vi "Signal Append.vi"() -> ()   [LabVIEW 2013]
panel:
  out "Flow":dynamicdata(graph)
  out "Audio":dynamicdata(graph)
  out "Pressure":dynamicdata(graph)
  out "Full Graph":dynamicdata(graph)
  out "SPL":dynamicdata(graph)
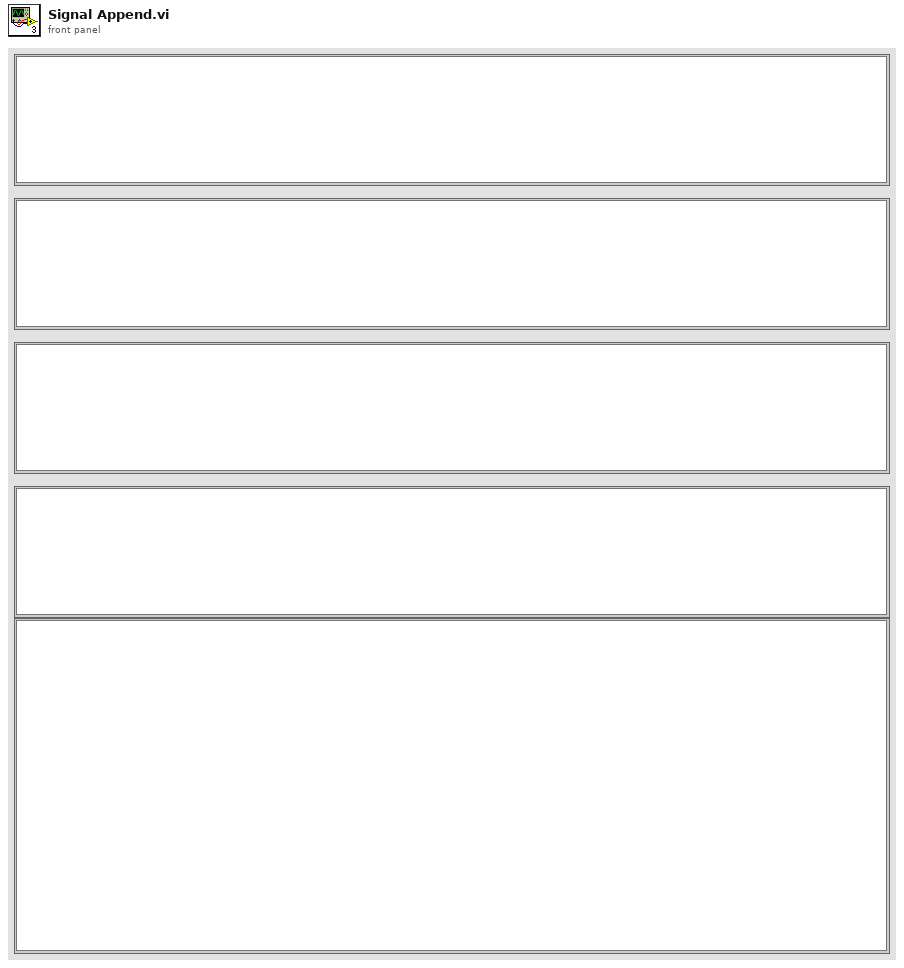
[diagram p1: front panel]
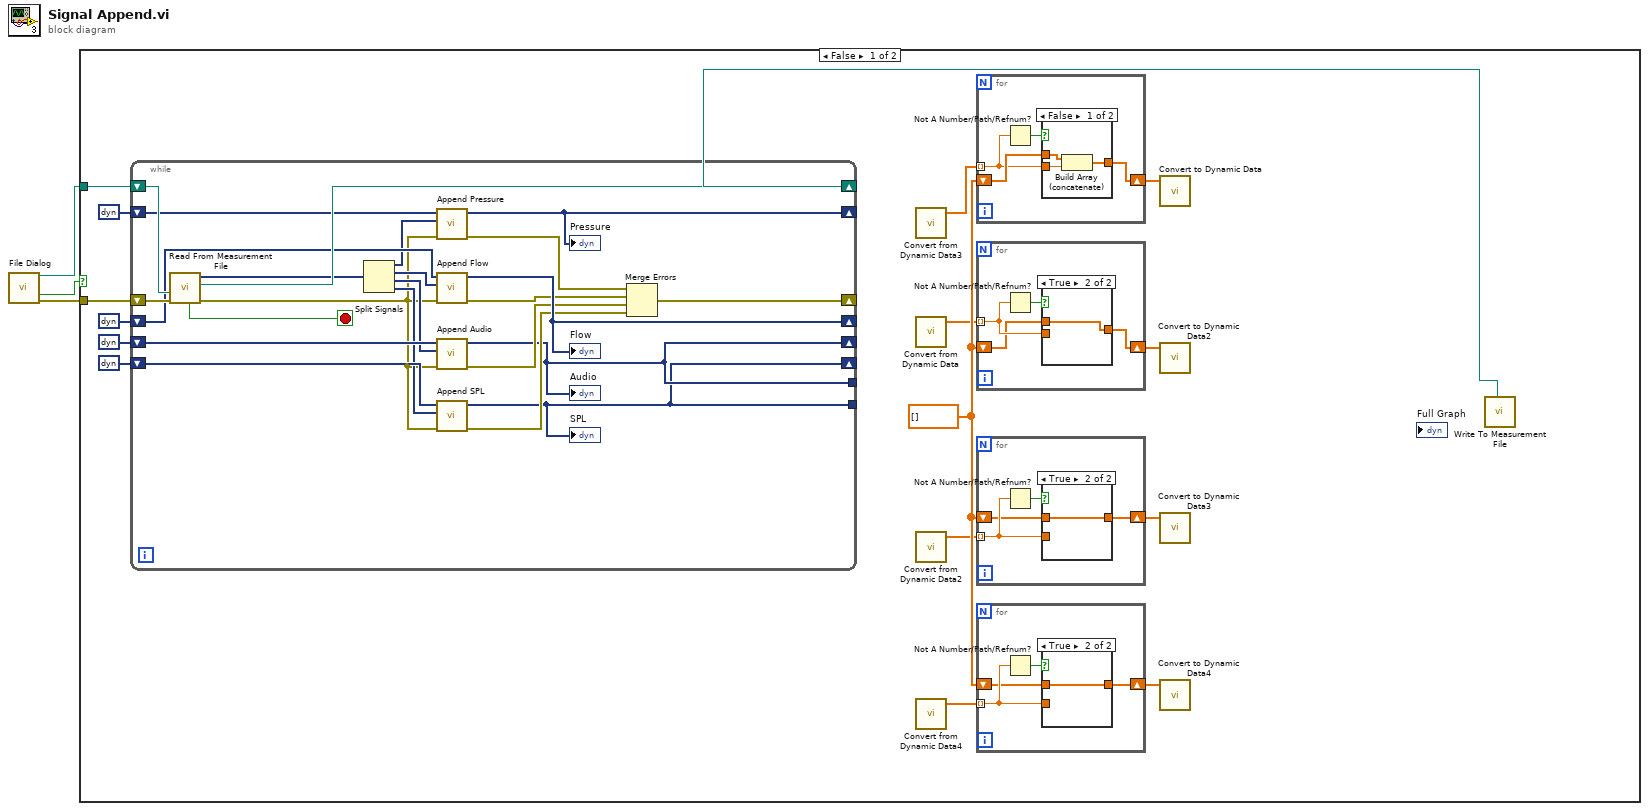
[diagram p0: block diagram]
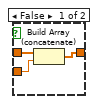
[diagram p2: hidden frame]
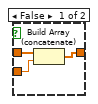
[diagram p3: hidden frame]
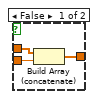
[diagram p4: hidden frame]
diagram:
  n1 = call "File Dialog"() -> ("selected path"=w3:path, "cancelled"=w1:bool, "error out"=w2:errorcluster)  [unwired: 12 in, 1 out]
  n2 = case shown="False" w1 {
    tunnel: w3 -> [w19 _]
    tunnel: w2 -> [w18 _]
    frame False {
      w7 = dbl[] [] ("Arrayin 2")
      n3 = while {
        shift-right: [w60] -> _
        shift-left: w18 -> [w73]
        shift-right: [w74] -> w13
        shift-left: w19 -> [w72]
        shift-right: [w63] -> _
        shift-left: dynamicdata [] ("Waveform Graph") -> [w70]
        shift-right: [w62] -> _
        shift-left: dynamicdata [] ("Waveform Graph") -> [w69]
        shift-right: [w53] -> _
        shift-left: dynamicdata [] ("Waveform Graph") -> [w68]
        shift-right: [w52] -> _
        shift-left: dynamicdata [] ("Waveform Graph") -> [w67]
        tunnel: [w53] -> _
        tunnel: [w52] -> _
        stop <- w71 stop-if-true
        n4 = call "Read From Measurement File"("error in (no error)"=w73, "Filename"=w72) -> ("error out"=w55:errorcluster, "Filename Out"=w74:path, "Signals"=w54:dynamicdata, "EOF?"=w71:bool)  [unwired: 4 in, 2 out]
        n5 = Split Signals(w54) -> (w66:dynamicdata, w65:dynamicdata, w64:dynamicdata, w61:dynamicdata)  [unwired: 4 in]
        n6 = call "Append Pressure"("error in (no error)"=w55, "Input Signal B"=w66, "Input Signal A"=w70) -> ("error out"=w59:errorcluster, "Appended Signals"=w63:dynamicdata)  [unwired: 7 in]
        "Pressure" <- w63
        n7 = call "Append Flow"("error in (no error)"=w55, "Input Signal B"=w65, "Input Signal A"=w69) -> ("error out"=w58:errorcluster, "Appended Signals"=w62:dynamicdata)  [unwired: 7 in]
        "Flow" <- w62
        n8 = call "Append Audio"("error in (no error)"=w55, "Input Signal B"=w64, "Input Signal A"=w68) -> ("error out"=w57:errorcluster, "Appended Signals"=w53:dynamicdata)  [unwired: 7 in]
        "Audio" <- w53
        n9 = call "Append SPL"("error in (no error)"=w55, "Input Signal B"=w61, "Input Signal A"=w67) -> ("error out"=w56:errorcluster, "Appended Signals"=w52:dynamicdata)  [unwired: 7 in]
        "SPL" <- w52
        n10 = Merge Errors(w59, w58, w57, w56) -> (w60:errorcluster)
      }
      n11 = call "Convert from Dynamic Data3"() -> ("Array"=w12:dbl[])  [unwired: 4 in]
      n12 = call "Convert from Dynamic Data"() -> ("Array"=w6:dbl[])  [unwired: 4 in]
      n13 = call "Convert from Dynamic Data2"() -> ("Array"=w5:dbl[])  [unwired: 4 in]
      n14 = call "Convert from Dynamic Data4"() -> ("Array"=w4:dbl[])  [unwired: 4 in]
      n15 = for {
        tunnel: w12 -> [w44] mode=indexing
        shift-right: [w45] -> w11
        shift-left: w7 -> [w46]
        n16 = Not A Number/Path/Refnum?(number/path/refnum=w44) -> (NaN/Path/Refnum?=w47:bool)
        n17 = case shown="False" w47 {
          tunnel: w46 -> [w50 w51]
          tunnel: [w49 w51] -> w45
          tunnel: w44 -> [w48 _]
          frame False {
            n18 = Build Array (concatenate)(w50, w48) -> (w49:dbl[])
          }
          frame True {
          }
        }
      }
      n19 = for {
        tunnel: w6 -> [w38] mode=indexing
        shift-right: [w36] -> w10
        shift-left: w7 -> [w37]
        n20 = Not A Number/Path/Refnum?(number/path/refnum=w38) -> (NaN/Path/Refnum?=w39:bool)
        n21 = case shown="True" w39 {
          tunnel: w37 -> [w42 w43]
          tunnel: [w41 w43] -> w36
          tunnel: w38 -> [w40 _]
          frame False {
            n22 = Build Array (concatenate)(w42, w40) -> (w41:dbl[])
          }
          frame True {
          }
        }
      }
      n23 = for {
        tunnel: w5 -> [w30] mode=indexing
        shift-right: [w28] -> w8
        shift-left: w7 -> [w29]
        n24 = Not A Number/Path/Refnum?(number/path/refnum=w30) -> (NaN/Path/Refnum?=w31:bool)
        n25 = case shown="True" w31 {
          tunnel: w29 -> [w34 w35]
          tunnel: [w33 w35] -> w28
          tunnel: w30 -> [w32 _]
          frame False {
            n26 = Build Array (concatenate)(w34, w32) -> (w33:dbl[])
          }
          frame True {
          }
        }
      }
      n27 = for {
        tunnel: w4 -> [w22] mode=indexing
        shift-right: [w20] -> w9
        shift-left: w7 -> [w21]
        n28 = Not A Number/Path/Refnum?(number/path/refnum=w22) -> (NaN/Path/Refnum?=w23:bool)
        n29 = case shown="True" w23 {
          tunnel: w21 -> [w26 w27]
          tunnel: [w25 w27] -> w20
          tunnel: w22 -> [w24 _]
          frame False {
            n30 = Build Array (concatenate)(w26, w24) -> (w25:dbl[])
          }
          frame True {
          }
        }
      }
      n31 = call "Convert to Dynamic Data"("Array"=w11) -> ()  [unwired: 3 in, 1 out]
      n32 = call "Convert to Dynamic Data2"("Array"=w10) -> ()  [unwired: 3 in, 1 out]
      n33 = call "Convert to Dynamic Data3"("Array"=w8) -> ()  [unwired: 3 in, 1 out]
      n34 = call "Convert to Dynamic Data4"("Array"=w9) -> ()  [unwired: 3 in, 1 out]
      n35 = call "Write To Measurement File"("Filename"=w13) -> ()  [unwired: 16 in, 3 out]
    }
    frame True {
    }
  }
